vi "GetMessage.vi"(8 "error in (no error)":errorcluster, 11 "TCP_Server_Connection_Handler in":refnum<class "TCP_Server_Connection_Handler.lvclass">) -> (0 "error out":errorcluster, 3 "TCP_Server_Connection_Handler out":refnum<class "TCP_Server_Connection_Handler.lvclass">)   [LabVIEW 2023, in "TCP_Server_Connection_Handler.lvlib" / "TCP_Server_Connection_Handler.lvclass"]
uses:
  TCP_Server_Connection_Handler.lvclass
  C:/Program Files (x86)/National Instruments/LabVIEW 2023/vi.lib/ActorFramework/Actor/Actor.lvclass
  TCP_Server_Connection_Handler.lvclass/TCP_Server_Connection_Handler.ctl
  <vilib>/ActorFramework/Actor/Actor.lvclass/Actor.ctl
  <vilib>/ActorFramework/Message Enqueuer/Message Enqueuer.lvclass/Message Enqueuer.ctl
  TCP_Server_Connection_Handler Messages/SaveFile Msg/SaveFile Msg.lvclass/SaveFile Msg.ctl
  <vilib>/ActorFramework/Message Enqueuer/Init from Existing Queue.vi
  <vilib>/ActorFramework/Message Enqueuer/Enqueue.vi
  TCP_Server_Connection_Handler Messages/SendMessageToCaller Msg/SendMessageToCaller Msg.lvclass
  C:/Program Files (x86)/National Instruments/LabVIEW 2023/vi.lib/ActorFramework/Message/Message.lvclass
  TCP_Server_Connection_Handler Messages/SaveFile Msg/SaveFile Msg.lvclass
  TCP_Server_Connection_Handler Messages/FindMessageStart Msg/FindMessageStart Msg.lvclass
  <vilib>/ActorFramework/Stop Msg/Stop Msg.lvclass
  <vilib>/ActorFramework/Message Priority Queue/Priority Enqueue.vi
  <vilib>/ActorFramework/Message Enqueuer/Message Enqueuer.lvclass
  <vilib>/ActorFramework/Actor/Actor.lvclass
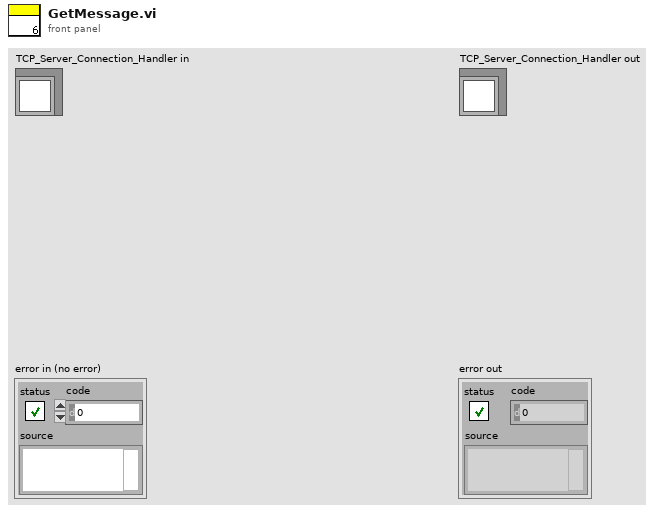
[diagram p1: front panel]
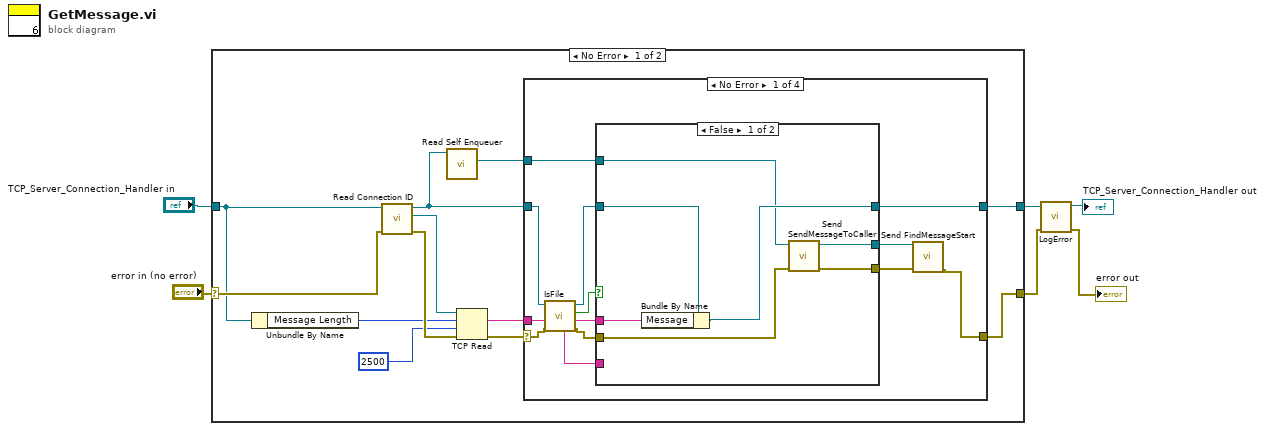
[diagram p0: block diagram]
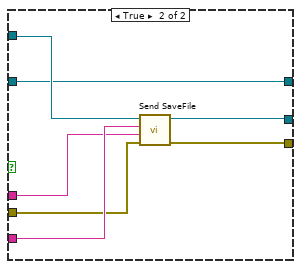
[diagram p2: hidden frame]
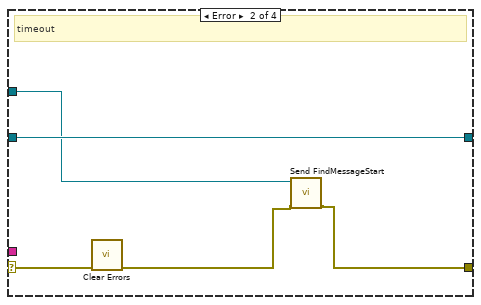
[diagram p3: hidden frame]
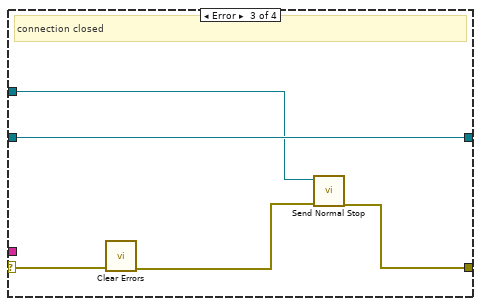
[diagram p4: hidden frame]
diagram:
  n1 = case shown="No Error" "error in (no error)" {
    selector: "error in (no error)" -> [w18 w59]
    tunnel: [w9 w59] -> w2
    tunnel: [w10 w58] -> w4
    tunnel: "TCP_Server_Connection_Handler in" -> [w15 w58]
    frame No Error {
      n2 = Unbundle By Name(w15) -> ("Message Length"=w14:i32)
      n3 = call "Read Connection ID.vi"("error in (no error)"=w18, "TCP_Server_Connection_Handler in"=w15) -> ("error out"=w16:errorcluster, "Connection ID"=w17:refnum<k5>, "TCP_Server_Connection_Handler out"=w8:refnum<class "TCP_Server_Connection_Handler.lvclass">)  [unwired: 7 in]
      n4 = call <vilib>:"Read Self Enqueuer.vi"("Actor"=w8) -> ("Self Enqueuer"=w7:refnum<class "Message Enqueuer.lvclass">)  [unwired: 10 in]
      n5 = TCP Read(connection ID=w17, bytes to read=w14, error in (no error)=w16, 9:2500 ("timeout ms (25000)")) -> (data out=w11:string, error out=w12:errorcluster)  [unwired: 1 in, 1 out]
      n6 = case shown="No Error" w12 {
        selector: w12 -> [w24 w48 w52 w56]
        tunnel: w11 -> [w26 _ _ _]
        tunnel: w8 -> [w22 w50 w55 w57]
        tunnel: [w31 w50 w55 w57] -> w10
        tunnel: [w27 w46 w53 w56] -> w9
        tunnel: w7 -> [w30 w49 w54 _]
        frame No Error {
          n7 = call "IsFile.vi"("error in (no error)"=w24, "message in"=w26, "TCP_Server_Connection_Handler in"=w22) -> ("error out"=w23:errorcluster, "message out"=w25:string, "IsFile?"=w19:bool, "TCP_Server_Connection_Handler out"=w21:refnum<class "TCP_Server_Connection_Handler.lvclass">, "Filename"=w20:string)  [unwired: 4 in]
          n8 = case shown="False" w19 {
            tunnel: w21 -> [w38 w39]
            tunnel: [w36 w39] -> w31
            tunnel: w30 -> [w35 w45]
            tunnel: w23 -> [w34 w42]
            tunnel: [w33 w40] -> w29
            tunnel: [w32 w41] -> w28
            tunnel: w20 -> [_ w44]
            tunnel: w25 -> [w37 w43]
            frame False {
              n9 = Bundle By Name(cluster=w38, "Message"=w37) -> (w36:refnum<class "TCP_Server_Connection_Handler.lvclass">)
              n10 = call "Send SendMessageToCaller.vi"("error in (no error)"=w34, "Message Enqueuer"=w35) -> ("error out"=w32:errorcluster, "Message Enqueuer out"=w33:refnum<class "Message Enqueuer.lvclass">)  [unwired: 8 in]
            }
            frame True {
              n11 = call "Send SaveFile.vi"("error in (no error)"=w42, "Data"=w43, "Filename"=w44, "Message Enqueuer"=w45) -> ("error out"=w41:errorcluster, "Message Enqueuer out"=w40:refnum<class "Message Enqueuer.lvclass">)  [unwired: 6 in]
            }
          }
          n12 = call "Send FindMessageStart.vi"("error in (no error)"=w28, "Message Enqueuer"=w29) -> ("error out"=w27:errorcluster)  [unwired: 8 in, 1 out]
        }
        frame Error {
          # "timeout"
          n13 = call <vilib>:"Clear Errors.vi"("error in (no error)"=w48) -> ("error out"=w47:errorcluster)  [unwired: 5 in, 1 out]
          n14 = call "Send FindMessageStart.vi"("error in (no error)"=w47, "Message Enqueuer"=w49) -> ("error out"=w46:errorcluster)  [unwired: 8 in, 1 out]
        }
        frame Error {
          # "connection closed"
          n15 = call <vilib>:"Clear Errors.vi"("error in (no error)"=w52) -> ("error out"=w51:errorcluster)  [unwired: 5 in, 1 out]
          n16 = call <vilib>:"Send Normal Stop.vi"("error in (no error)"=w51, "Message Enqueuer"=w54) -> ("error out"=w53:errorcluster)  [unwired: 9 in]
        }
        frame Default {
        }
      }
    }
    frame Error {
    }
  }
  n17 = call "LogError.vi"("error in (no error)"=w2, "TCP_Server_Connection_Handler in"=w4) -> ("error out"=→"error out":errorcluster, "TCP_Server_Connection_Handler out"=→"TCP_Server_Connection_Handler out":refnum<class "TCP_Server_Connection_Handler.lvclass">)  [unwired: 8 in]
